vi "edit exit.vi"(0 "appended path":path, 1 "error in (no error)":errorcluster, 4 "genneral info":string, 5 "path":path, 6 "保存":refnum<vi>, 7 "Edit":bool, 8 "Ready":refnum<vi>, 9 "tpdata":string[](array[string]), 10 "Program Name:":refnum<vi>, 11 "TP Information":refnum<vi>) -> (2 "error out":errorcluster, 3 "布尔":bool)   [LabVIEW 2018]
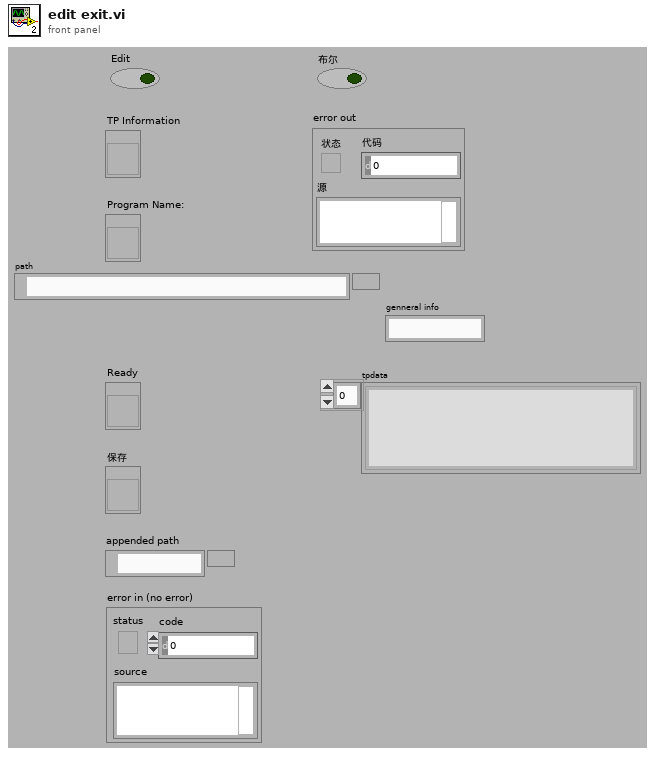
[diagram p1: front panel]
types:
  T1 = enum16{"open", "replace", "create", "open or create", "replace or create", "replace or create with confirmation"}
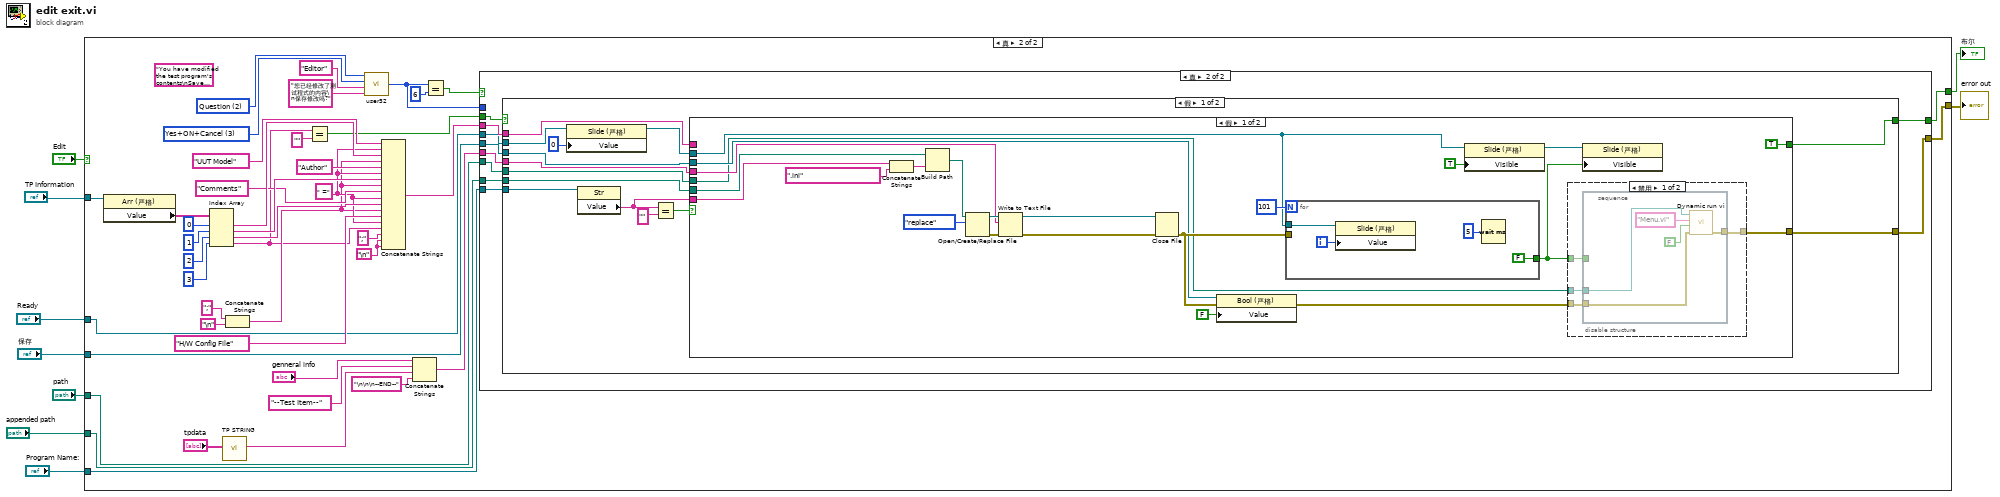
[diagram p0: block diagram]
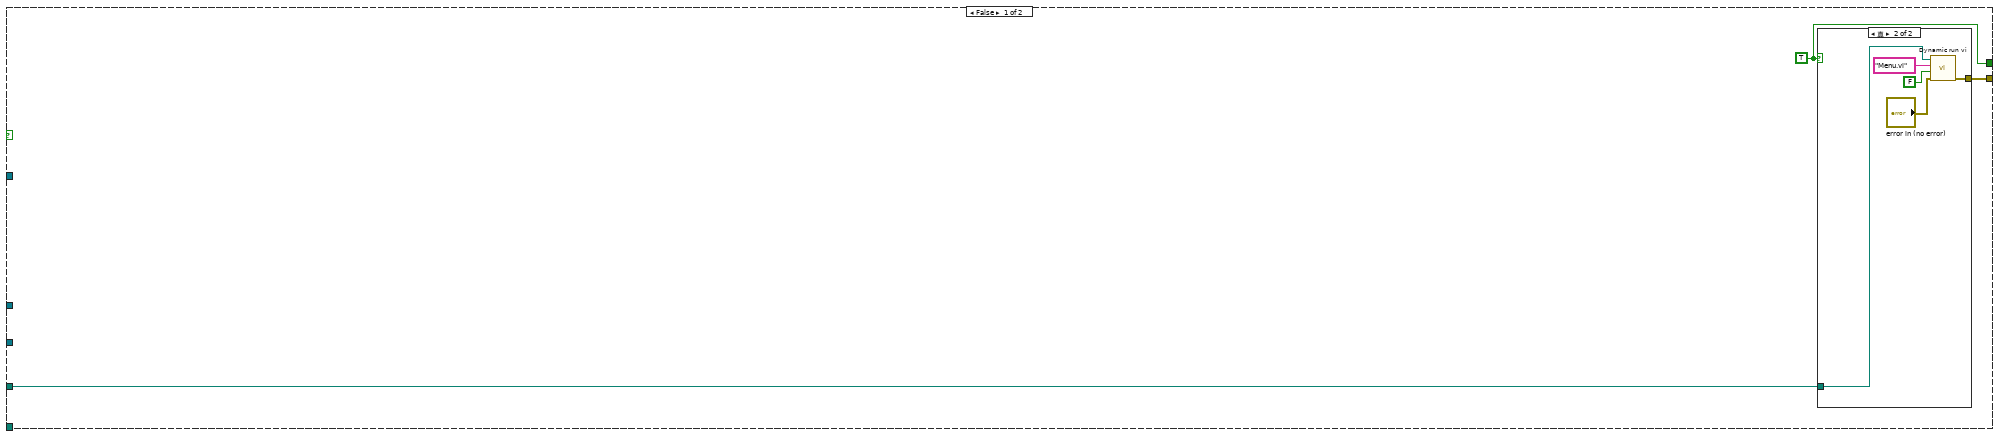
[diagram p2: hidden frame]
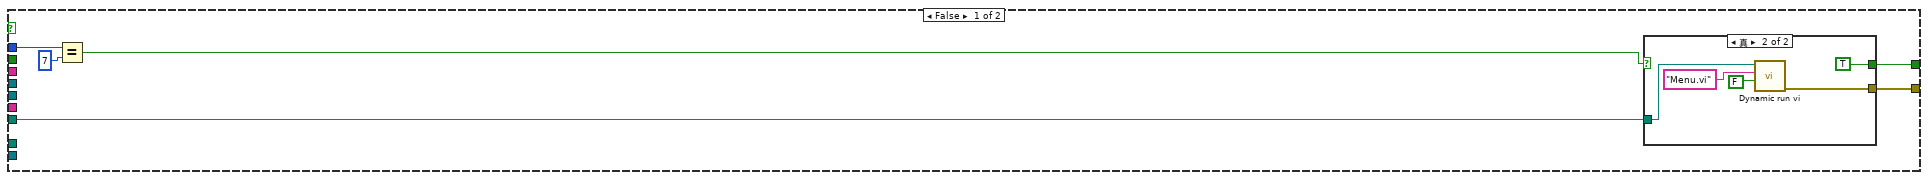
[diagram p4: hidden frame]
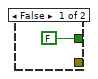
[diagram p5: hidden frame]
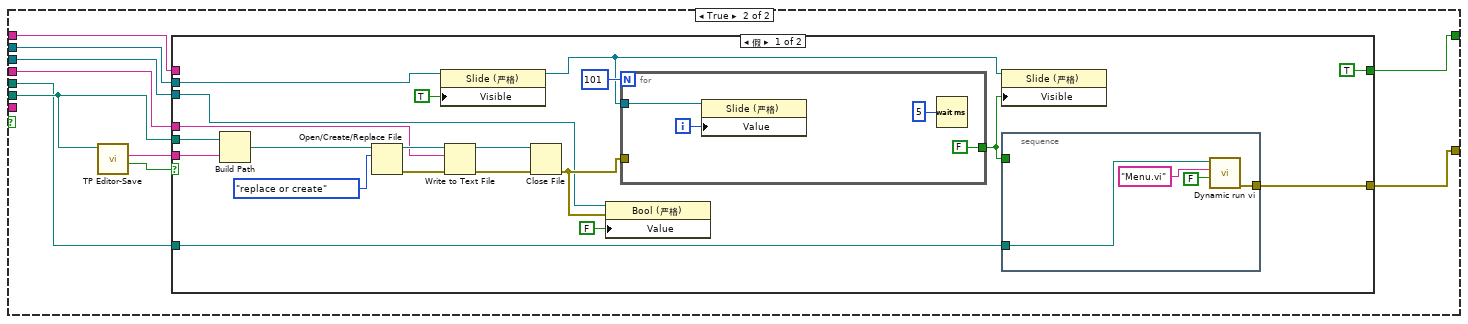
[diagram p7: hidden frame]
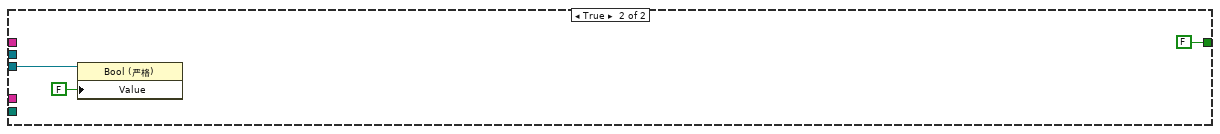
[diagram p8: hidden frame]
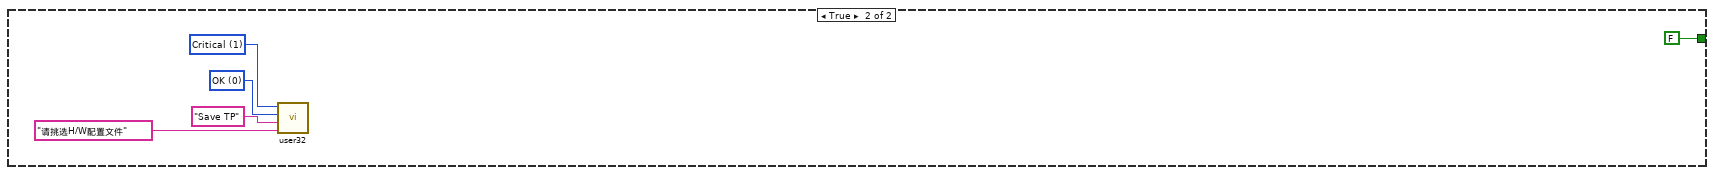
[diagram p9: hidden frame]
diagram:
  n1 = case shown="真" "Edit" {
    tunnel: [w12 w53] -> w6
    tunnel: [w11 w52] -> w7
    tunnel: "appended path" -> [_ w55]
    tunnel: "TP Information" -> [_ w29]
    tunnel: "Program Name:" -> [_ w28]
    tunnel: "保存" -> [_ w26]
    tunnel: "Ready" -> [_ w27]
    tunnel: "path" -> [w10 w18]
    frame False {
      w11 = TRUE
      n2 = case shown="真" w11 {
        tunnel: [_ w15] -> w12
        tunnel: w10 -> [_ w13]
        frame False {
        }
        frame True {
          n3 = call "Dynamic run vi.vi"("error in (no error)"="error in (no error)", "Wait Until Done"=FALSE, "vi name"="Menu.vi", "path"=w13) -> ("error out"=w15:errorcluster)  [unwired: 4 out]
        }
      }
    }
    frame True {
      w37 = "\n"
      w40 = " ="
      (unwired) "You have modified the test program's contents\nSave changes?" ("IP Text")
      w59 = u16 3 items=["OK", "OK+Cancel", "Abort+Retry+Ignore", "Yes+ON+Cancel", "Yes+No", "Retry+Cancel", "Cancel+Retry+Continue"] ("Buttons")
      w60 = u16 2 items=["None", "Critical", "Question", "Exclamation", "Infomation"] ("Icon")
      n4 = property on="属性节点" class="Arr (严格)"(reference=w29) -> ("Value"=w32:string[])  [unwired: 1 in, 2 out]
      n5 = Index Array(array=w32, index #1=0 ("index"), index #2=1 ("index"), index #3=2 ("index"), index #4=3 ("index")) -> (element #1=w46:string, element #2=w44:string, element #3=w42:string, element #4=w34:string)
      n6 = call "TP STRING.vi"("tpdata"="tpdata") -> ("TP OUT"=w23:string)  [unwired: 1 in, 9 out]
      n7 = Concatenate Strings(";" ("string"), "\n") -> (w39:string)
      n8 = Equal?(x=w34, y="") -> (x = y?=w30:bool)
      n9 = call "user32.vi"("Icon"=w60, "Buttons"=w59, "Ipcaption"="Editor", "IP Text"="您已经修改了测试程式的内容\n保存修改吗?") -> ("buttin pressed"=w54:i32)  [unwired: 1 out]
      n10 = Concatenate Strings("UUT Model", w40, w46, w39, "Author", w40, w44, w39, "Comments", w40, w42, w39, "H/W Config File", w40, w34, ";", w37, w37) -> (w31:string)
      n11 = Concatenate Strings("genneral info", "--Test Item--" ("字符串"), w23, "\n\n\n--END--") -> (w20:string)
      n12 = Equal?(x=w54, y=6) -> (x = y?=w56:bool)
      n13 = case shown="真" w56 {
        tunnel: w55 -> [_ w82]
        tunnel: w54 -> [w66 _]
        tunnel: [w64 w80] -> w53
        tunnel: [w62 w81] -> w52
        tunnel: w31 -> [_ w79]
        tunnel: w30 -> [_ w78]
        tunnel: w28 -> [_ w77]
        tunnel: w26 -> [_ w76]
        tunnel: w27 -> [_ w75]
        tunnel: w20 -> [_ w74]
        tunnel: w18 -> [w61 w73]
        frame False {
          n14 = Equal?(x=w66, y=7) -> (x = y?=w63:bool)
          n15 = case shown="真" w63 {
            tunnel: [_ w70] -> w64
            tunnel: [FALSE TRUE] -> w62
            tunnel: w61 -> [_ w68]
            frame False {
            }
            frame True {
              n16 = call "Dynamic run vi.vi"("Wait Until Done"=FALSE, "vi name"="Menu.vi", "path"=w68) -> ("error out"=w70:errorcluster)  [unwired: 1 in, 4 out]
            }
          }
        }
        frame True {
          n17 = case shown="假" w78 {
            tunnel: w82 -> [w92 _]
            tunnel: [w91 FALSE] -> w81
            tunnel: [w90 _] -> w80
            tunnel: w79 -> [w89 _]
            tunnel: w77 -> [w88 _]
            tunnel: w76 -> [w86 _]
            tunnel: w75 -> [w87 _]
            tunnel: w74 -> [w84 _]
            tunnel: w73 -> [w83 _]
            frame False {
              n18 = property on="属性节点" class="Slide (严格)"(reference=w87, "Value"=0) -> (reference out=w85:refnum<vi>)  [unwired: 1 in, 1 out]
              n19 = property on="属性节点" class="Str"(reference=w88) -> ("Value"=w94:string)  [unwired: 1 in, 2 out]
              n20 = Equal?(x=w94, y="") -> (x = y?=w95:bool)
              n21 = case shown="假" w95 {
                tunnel: w94 -> [w117 _]
                tunnel: w92 -> [w118 w141]
                tunnel: [TRUE w139] -> w91
                tunnel: [w103 w138] -> w90
                tunnel: w89 -> [_ w137]
                tunnel: w85 -> [w100 w135]
                tunnel: w86 -> [w99 w136]
                tunnel: w84 -> [w98 w134]
                tunnel: w83 -> [w97 w133]
                frame False {
                  n22 = Concatenate Strings(w117, ".ini") -> (w115:string)
                  n23 = Build Path(base path=w118, name or relative path=w115) -> (appended path=w119:path)
                  n24 = Open/Create/Replace File(file path (use dialog)=w119, operation (0:open)=T1."replace") -> (refnum out=w106:refnum<file>, error out=w107:errorcluster)  [unwired: 1 in, 4 out]
                  n25 = Write to Text File(file (use dialog)=w106, text=w98, error in=w107) -> (refnum out=w113:refnum<file>, error out=w112:errorcluster)  [unwired: 2 out]
                  n26 = Close File(refnum=w113, error in=w112) -> (error out=w108:errorcluster)  [unwired: 1 out]
                  n27 = property on="属性节点" class="Bool (严格)"(reference=w99, error in=w108, "Value"=FALSE) -> (error out=w104:errorcluster)  [unwired: 1 out]
                  n28 = for {
                    N: 101 -> [_]
                    tunnel: [FALSE] -> w102
                    tunnel: w108 -> [_]
                    tunnel: w100 -> [w129]
                    i -> [w132]
                    n29 = property on="属性节点" class="Slide (严格)"(reference=w129, "Value"=w132) -> ()  [unwired: 1 in, 2 out]
                    n30 = Wait (ms)(milliseconds to wait=u32 5) -> ()  [unwired: 1 out]
                  }
                  n31 = property on="属性节点" class="Slide (严格)"(reference=w100, "Visible"=TRUE) -> (reference out=w101:refnum<vi>)  [unwired: 1 in, 1 out]
                  n32 = disable-structure shown="禁用" {
                    disable-tunnel: w104 -> [w123 _]
                    disable-tunnel: [w122 _] -> w103
                    disable-tunnel: w102 -> [w121 _]
                    disable-tunnel: w97 -> [w120 _]
                    frame Disabled {
                      n33 = stacked-sequence {
                        tunnel: w123 -> [w126]
                        tunnel: [w125] -> w122
                        tunnel: w121 -> [_]
                        tunnel: w120 -> [w124]
                        frame #0 {
                          n34 = call "Dynamic run vi.vi"("error in (no error)"=w126, "Wait Until Done"=FALSE, "vi name"="Menu.vi", "path"=w124) -> ("error out"=w125:errorcluster)  [unwired: 4 out]
                        }
                      }
                    }
                    frame Enabled {
                    }
                  }
                  n35 = property on="属性节点" class="Slide (严格)"(reference=w101, "Visible"=w102) -> ()  [unwired: 1 in, 2 out]
                }
                frame True {
                  n36 = call "TP Editor-Save.vi"("path"=w141) -> ("Cancel"=w140:bool, "File Name 2"=w142:string)  [unwired: 1 in, 5 out]
                  n37 = case shown="假" w140 {
                    tunnel: w142 -> [w159 _]
                    tunnel: w141 -> [w157 _]
                    tunnel: [TRUE FALSE] -> w139
                    tunnel: [w150 _] -> w138
                    tunnel: w137 -> [_ _]
                    tunnel: w135 -> [w147 _]
                    tunnel: w136 -> [w146 w171]
                    tunnel: w134 -> [w144 _]
                    tunnel: w133 -> [w143 _]
                    frame False {
                      n38 = Build Path(base path=w157, name or relative path=w159) -> (appended path=w162:path)
                      n39 = Open/Create/Replace File(file path (use dialog)=w162, operation (0:open)=T1."replace or create") -> (refnum out=w161:refnum<file>, error out=w160:errorcluster)  [unwired: 1 in, 4 out]
                      n40 = property on="属性节点" class="Slide (严格)"(reference=w147, "Visible"=TRUE) -> (reference out=w145:refnum<vi>)  [unwired: 1 in, 1 out]
                      n41 = Write to Text File(file (use dialog)=w161, text=w144, error in=w160) -> (refnum out=w153:refnum<file>, error out=w152:errorcluster)  [unwired: 2 out]
                      n42 = Close File(refnum=w153, error in=w152) -> (error out=w149:errorcluster)  [unwired: 1 out]
                      n43 = property on="属性节点" class="Bool (严格)"(reference=w146, error in=w149, "Value"=FALSE) -> ()  [unwired: 2 out]
                      n44 = for {
                        N: 101 -> [_]
                        tunnel: [FALSE] -> w148
                        tunnel: w149 -> [_]
                        tunnel: w145 -> [w163]
                        i -> [w166]
                        n45 = property on="属性节点" class="Slide (严格)"(reference=w163, "Value"=w166) -> ()  [unwired: 1 in, 2 out]
                        n46 = Wait (ms)(milliseconds to wait=u32 5) -> ()  [unwired: 1 out]
                      }
                      n47 = property on="属性节点" class="Slide (严格)"(reference=w145, "Visible"=w148) -> ()  [unwired: 1 in, 2 out]
                      n48 = stacked-sequence {
                        tunnel: [w168] -> w150
                        tunnel: w148 -> [_]
                        tunnel: w143 -> [w167]
                        frame #0 {
                          n49 = call "Dynamic run vi.vi"("Wait Until Done"=FALSE, "vi name"="Menu.vi", "path"=w167) -> ("error out"=w168:errorcluster)  [unwired: 1 in, 4 out]
                        }
                      }
                    }
                    frame True {
                      n50 = property on="属性节点" class="Bool (严格)"(reference=w171, "Value"=FALSE) -> ()  [unwired: 1 in, 2 out]
                    }
                  }
                }
              }
            }
            frame True {
              w177 = u16 0 items=["OK", "OK+Cancel", "Abort+Retry+Ignore", "Yes+ON+Cancel", "Yes+No", "Retry+Cancel", "Cancel+Retry+Continue"] ("Buttons")
              w178 = u16 1 items=["None", "Critical", "Question", "Exclamation", "Infomation"] ("Icon")
              n51 = call "user32.vi"("Icon"=w178, "Buttons"=w177, "Ipcaption"="Save TP", "IP Text"="请挑选H/W配置文件") -> ()  [unwired: 2 out]
            }
          }
        }
      }
    }
  }
  "布尔" <- w7
  "error out" <- w6
